vi "Compose TOML String.vi"(8 "error in (no error)":errorcluster, 11 "Value":T1) -> (0 "error out":errorcluster, 3 "String":string)   [LabVIEW 2017, in "TOML.lvlib"]
uses:
  TOML.lvlib
  TOML Value.ctl
  Compose Data.ctl
  Value.ctl
  Value Type.ctl
  Key-Value Pair.ctl
  <vilib>/ErrorRing/Error Ring.xnode
  <vilib>/regexp/Match Regular Expression.xnode
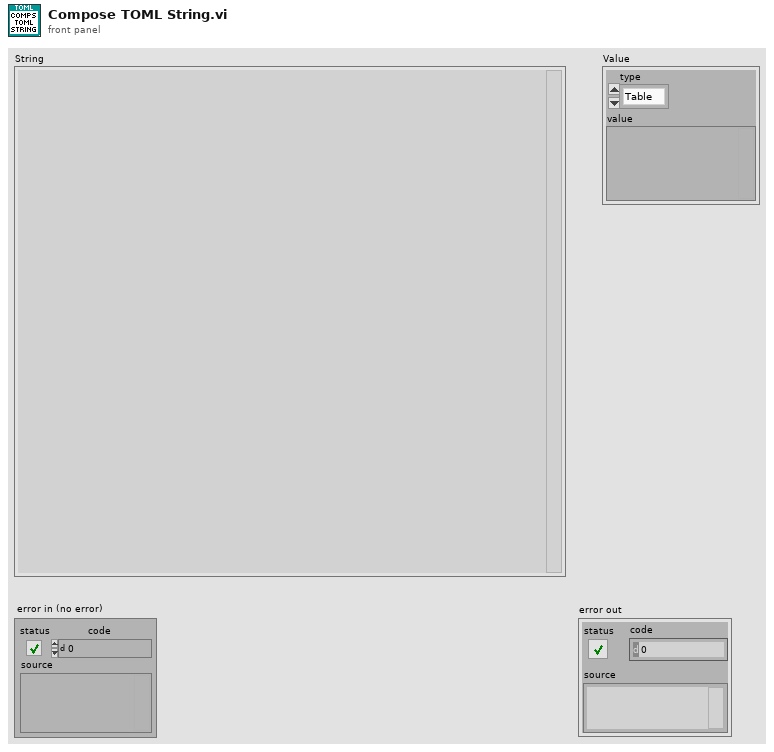
[diagram p1: front panel]
types:
  T1 = typedef "TOML.lvlib/TOML Value.ctl" = cluster{"type":enum16{"Table", "Array", "String", "Integer", "Float", "Boolean", "Offset Date-Time", "Local Date-Time", "Local Date", "Local Time", "Path"}, "value":variant}
  T2 = typedef "TOML.lvlib/Compose Data.ctl" = cluster{"Value":T3, "Prepend":string, "Append":string, "Inline":bool, "Name":string}
  T3 = typedef "TOML.lvlib/Value.ctl" = cluster{"Type":T4, "Value":variant}
  T4 = typedef "TOML.lvlib/Value Type.ctl" = enum16{"Table", "Array", "String", "Integer", "Float", "Boolean", "Offset Date-Time", "Local Date-Time", "Local Date", "Local Time", "Path"}
  T5 = typedef "TOML.lvlib/Key-Value Pair.ctl" = cluster{"Key":string, "Value":T3}
  T6 = enum16{"Table", "Array", "String", "Integer", "Float", "Boolean", "Offset Date-Time", "Local Date-Time", "Local Date", "Local Time"}
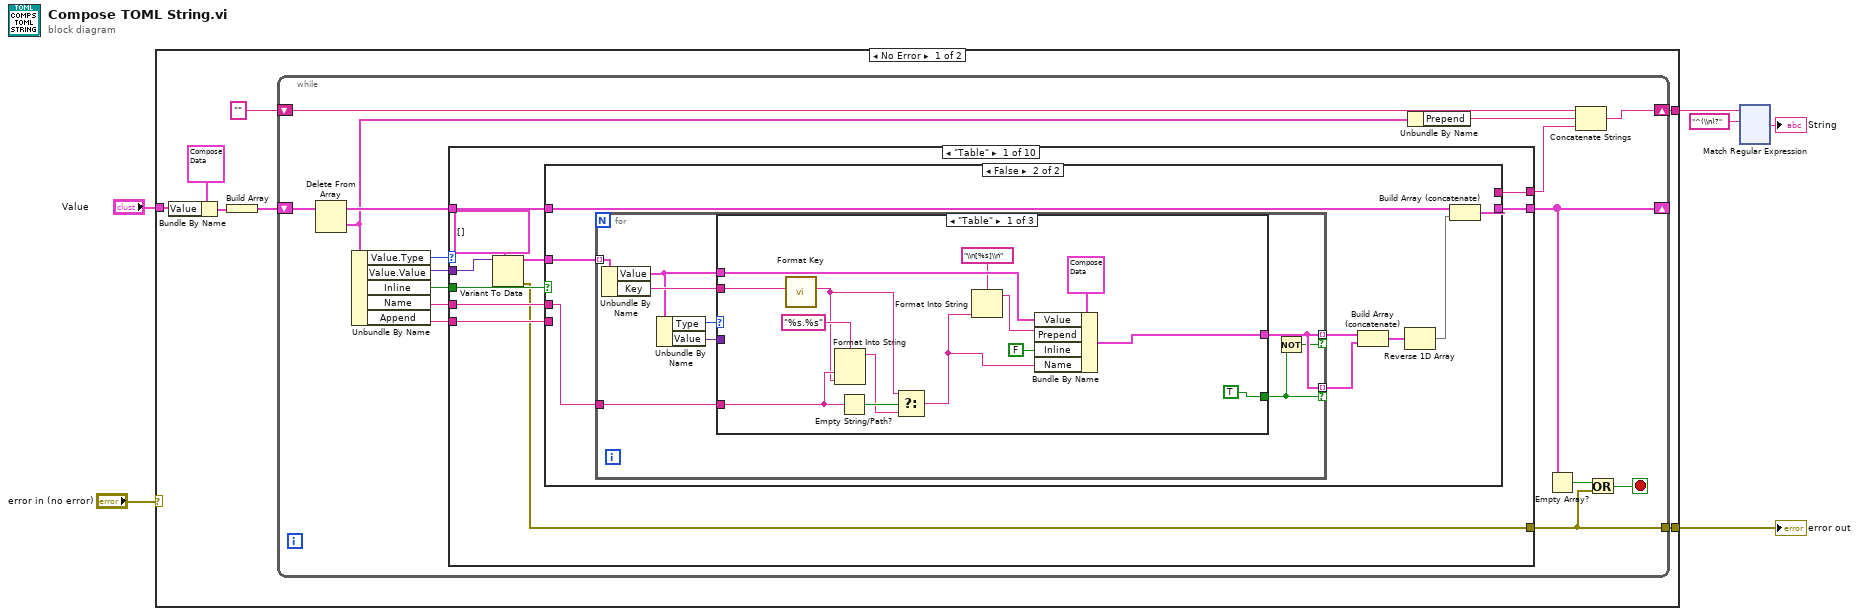
[diagram p0: block diagram]
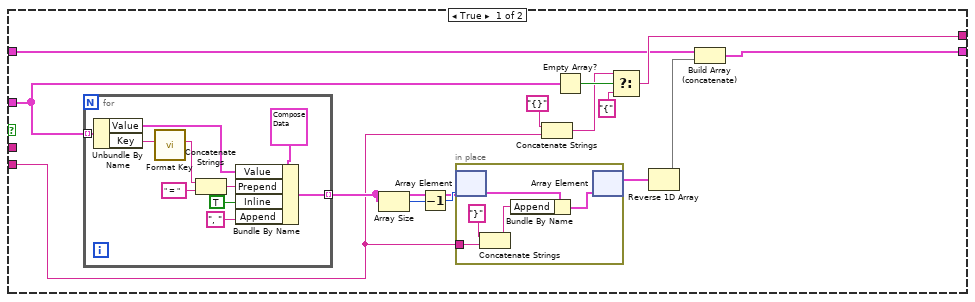
[diagram p2: hidden frame]
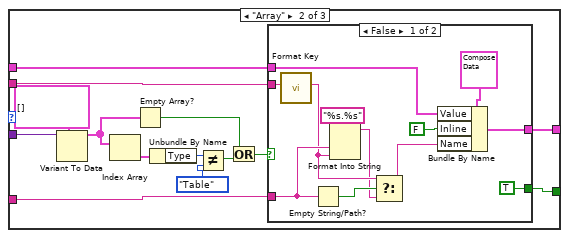
[diagram p3: hidden frame]
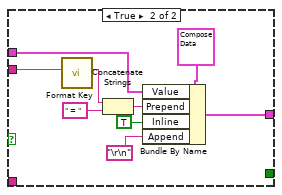
[diagram p4: hidden frame]
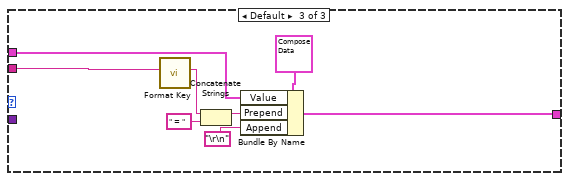
[diagram p5: hidden frame]
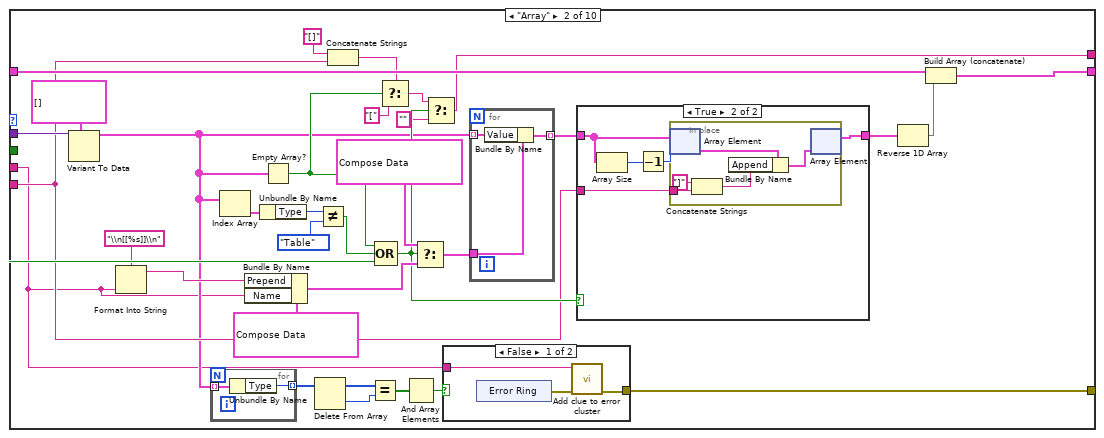
[diagram p6: hidden frame]
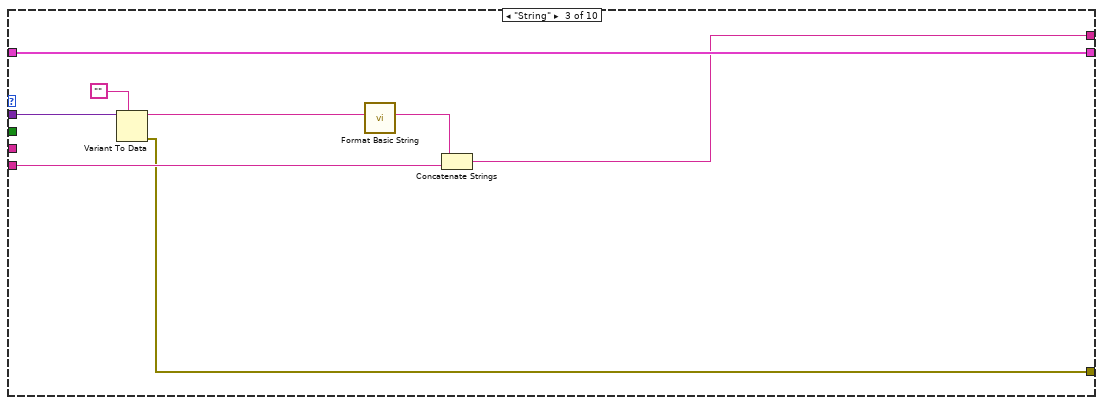
[diagram p9: hidden frame]
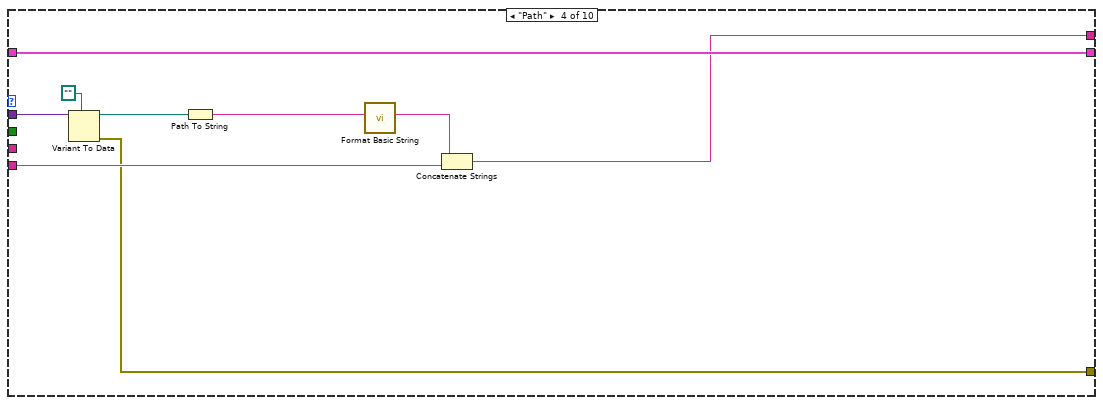
[diagram p10: hidden frame]
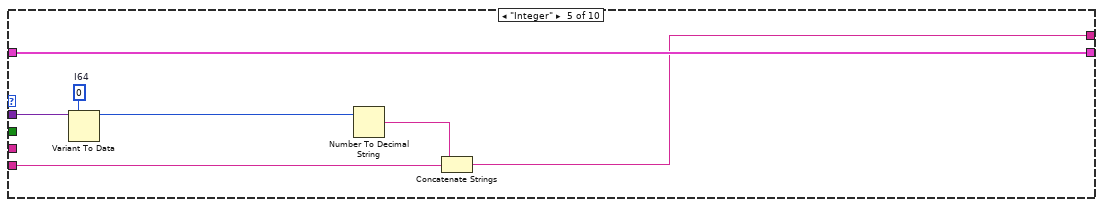
[diagram p11: hidden frame]
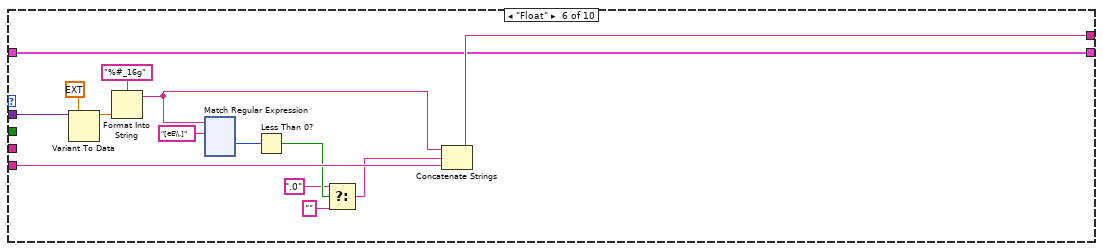
[diagram p12: hidden frame]
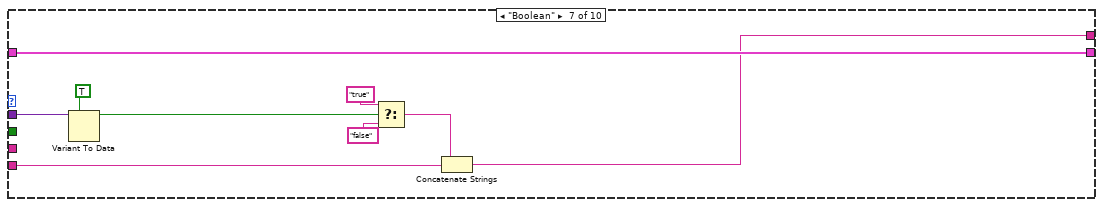
[diagram p13: hidden frame]
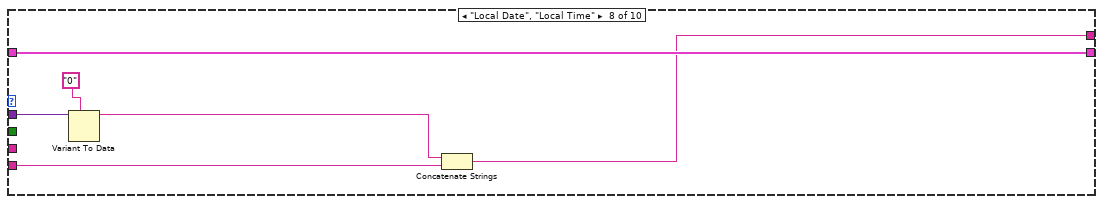
[diagram p14: hidden frame]
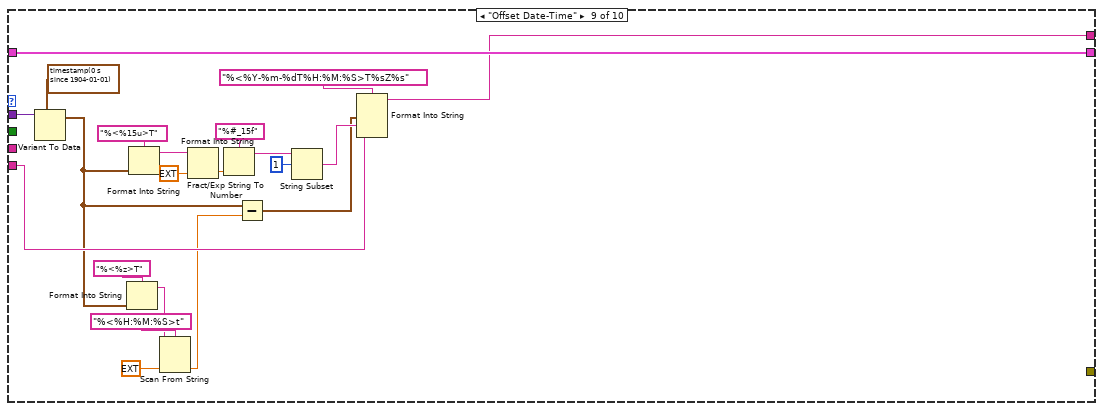
[diagram p15: hidden frame]
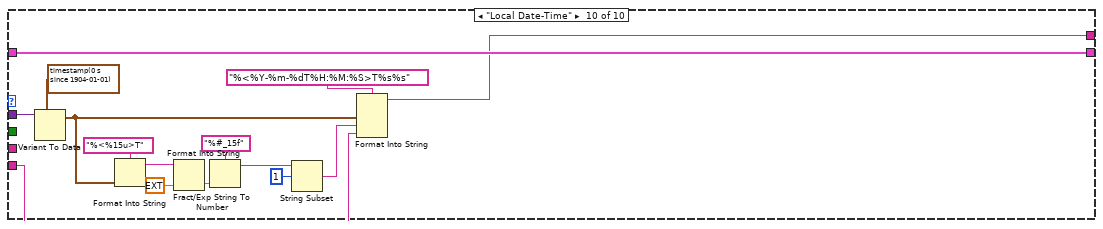
[diagram p16: hidden frame]
diagram:
  n1 = case shown="No Error" "error in (no error)" {
    selector: "error in (no error)" -> [_ w401]
    tunnel: "Value" -> [w10 _]
    tunnel: [w8 _] -> w1
    tunnel: [w7 w401] -> w4
    frame No Error {
      n2 = Bundle By Name(cluster=T2 {"Value"={"Type"=enum."Table", "Value"=variant}, "Prepend"="", "Append"="", "Inline"=FALSE, "Name"=""}, "Value"=w10) -> (w9:T2)
      n3 = Build Array(w9) -> (w12:T2[])
      n4 = while {
        shift-right: [w20] -> w8
        shift-left: "" -> [w23]
        shift-right: [w21] -> _
        shift-left: w12 -> [w29]
        tunnel: [w14] -> w7
        stop <- w15 stop-if-true
        n5 = Delete From Array(array=w29) -> (deleted portion=w18:T2, array with subset deleted=w26:T2[])  [unwired: 2 in]
        n6 = Unbundle By Name(w18) -> ("Value.Type"=w28:T4, "Value.Value"=w27:variant, "Inline"=w25:bool, "Name"=w24:string, "Append"=w16:string)
        n7 = case shown="\"Table\"" w28 {
          tunnel: w27 -> [w36 w177 w204 w213 w220 w235 w358 w364 w384 w399]
          tunnel: w26 -> [w39 w164 w205 w214 w221 w230 w356 w362 w385 w400]
          tunnel: [w38 w151 w205 w214 w221 w230 w356 w362 w385 w400] -> w21
          tunnel: w25 -> [w37 w171 _ _ _ _ _ _ _ _]
          tunnel: w24 -> [w31 w143 _ _ _ _ _ _ _ _]
          tunnel: [w32 w157 w200 w209 w215 w232 w350 w359 w376 w393] -> w19
          tunnel: w16 -> [w33 w152 w201 w210 w218 w233 w357 w363 w377 w394]
          tunnel: [w30 w145 w198 w206 _ _ _ _ _ _] -> w14
          frame "Table" {
            n8 = Variant To Data(type=T5[] [], Variant=w36) -> (data=w34:T5[], error out=w30:errorcluster)  [unwired: 1 in]
            n9 = case shown="False" w37 {
              tunnel: w39 -> [w43 w76]
              tunnel: [w42 w75] -> w38
              tunnel: w34 -> [w50 w72]
              tunnel: w31 -> [_ w74]
              tunnel: w33 -> [w47 _]
              tunnel: [w46 _] -> w32
              frame True {
                n10 = for {
                  tunnel: w50 -> [w68] mode=indexing
                  tunnel: [w60] -> w51 mode=indexing
                  n11 = Unbundle By Name(w68) -> ("Value"=w65:T3, "Key"=w67:string)
                  n12 = call "Format Key.vi"("Key String"=w67) -> ("Formatted Key"=w63:string)  [unwired: 10 in]
                  n13 = Concatenate Strings(w63, " = " ("string")) -> (w64:string)
                  n14 = Bundle By Name(cluster=T2 {"Value"={"Type"=enum."Table", "Value"=variant}, "Prepend"="", "Append"="", "Inline"=FALSE, "Name"=""}, "Value"=w65, "Prepend"=w64, "Inline"=TRUE, "Append"=", ") -> (w60:T2)
                }
                n15 = Array Size(array=w51) -> (size(s)=w53:i32)
                n16 = Decrement(x=w53) -> (x-1=w52:i32)
                n17 = in-place {
                  in-place-border: w47 -> [w54]
                  n18 = in-place-array #1(w51, w52) -> (w58:T2)
                  n19 = Concatenate Strings("}" ("Prepend"), w54) -> (w55:string)
                  n20 = Bundle By Name(cluster=w58, "Append"=w55) -> (w57:T2)
                  n21 = in-place-array #1(w57) -> (w45:T2[])  [unwired: 1 out]
                }
                n22 = Concatenate Strings("{}" ("Prepend"), w47) -> (w40:string)
                n23 = Empty Array?(array=w50) -> (empty?=w49:bool)
                n24 = Select(t=w40, s=w49, f="{" ("t")) -> (s? t:f=w46:string)
                n25 = Reverse 1D Array(array=w45) -> (reversed array=w44:T2[])
                n26 = Build Array (concatenate)(w43, w44) -> (w42:T2[])
              }
              frame False {
                n27 = for {
                  tunnel: w72 -> [w85] mode=indexing
                  tunnel: [w79] -> w70 mode=indexing if=w78
                  tunnel: w74 -> [w81]
                  tunnel: [w79] -> w69 mode=indexing if=w77
                  n28 = Unbundle By Name(w85) -> ("Value"=w83:T3, "Key"=w84:string)
                  n29 = Unbundle By Name(w83) -> ("Type"=w82:T4, "Value"=w80:variant)
                  n30 = case shown="\"Table\"" w82 {
                    tunnel: w84 -> [w99 w113 w138]
                    tunnel: [w96 w112 w135] -> w79
                    tunnel: w83 -> [w95 w111 w137]
                    tunnel: w81 -> [w91 w110 _]
                    tunnel: w80 -> [_ w102 _]
                    tunnel: [TRUE w100 _] -> w77
                    frame "Table" {
                      n31 = call "Format Key.vi"("Key String"=w99) -> ("Formatted Key"=w89:string)  [unwired: 10 in]
                      n32 = Format Into String(format string="%s.%s", w91, w89) -> (resulting string=w88:string)  [unwired: 2 in, 1 out]
                      n33 = Empty String/Path?(string/path=w91) -> (empty?=w90:bool)
                      n34 = Select(t=w89, s=w90, f=w88) -> (s? t:f=w87:string)
                      n35 = Format Into String(format string="\\n[%s]\\n", w87) -> (resulting string=w92:string)  [unwired: 2 in, 1 out]
                      n36 = Bundle By Name(cluster=T2 {"Value"={"Type"=enum."Table", "Value"=variant}, "Prepend"="", "Append"="", "Inline"=FALSE, "Name"=""}, "Value"=w95, "Prepend"=w92, "Inline"=FALSE, "Name"=w87) -> (w96:T2)
                    }
                    frame "Array" {
                      n37 = Variant To Data(type=T3[] [], Variant=w102) -> (data=w105:T3[])  [unwired: 1 in, 1 out]
                      n38 = Index Array(array=w105) -> (element=w107:T3)  [unwired: 1 in]
                      n39 = Empty Array?(array=w105) -> (empty?=w109:bool)
                      n40 = Unbundle By Name(w107) -> ("Type"=w106:T4)
                      n41 = Not Equal?(x=w106, y=T6."Table") -> (x != y?=w108:bool)
                      n42 = Or(x=w109, y=w108) -> (x .or. y?=w101:bool)
                      n43 = case shown="False" w101 {
                        tunnel: w113 -> [w120 w128]
                        tunnel: [w123 w126] -> w112
                        tunnel: w111 -> [w122 w129]
                        tunnel: w110 -> [w119 _]
                        tunnel: [TRUE _] -> w100
                        frame False {
                          n44 = call "Format Key.vi"("Key String"=w120) -> ("Formatted Key"=w117:string)  [unwired: 10 in]
                          n45 = Empty String/Path?(string/path=w119) -> (empty?=w118:bool)
                          n46 = Format Into String(format string="%s.%s", w119, w117) -> (resulting string=w116:string)  [unwired: 2 in, 1 out]
                          n47 = Select(t=w117, s=w118, f=w116) -> (s? t:f=w115:string)
                          n48 = Bundle By Name(cluster=T2 {"Value"={"Type"=enum."Table", "Value"=variant}, "Prepend"="", "Append"="", "Inline"=FALSE, "Name"=""}, "Value"=w122, "Inline"=FALSE, "Name"=w115) -> (w123:T2)
                        }
                        frame True {
                          n49 = call "Format Key.vi"("Key String"=w128) -> ("Formatted Key"=w132:string)  [unwired: 10 in]
                          n50 = Concatenate Strings(w132, " = " ("string")) -> (w133:string)
                          n51 = Bundle By Name(cluster=T2 {"Value"={"Type"=enum."Table", "Value"=variant}, "Prepend"="", "Append"="", "Inline"=FALSE, "Name"=""}, "Value"=w129, "Prepend"=w133, "Inline"=TRUE, "Append"="\r\n") -> (w126:T2)
                        }
                      }
                    }
                    frame Default {
                      n52 = call "Format Key.vi"("Key String"=w138) -> ("Formatted Key"=w140:string)  [unwired: 10 in]
                      n53 = Concatenate Strings(w140, " = " ("string")) -> (w141:string)
                      n54 = Bundle By Name(cluster=T2 {"Value"={"Type"=enum."Table", "Value"=variant}, "Prepend"="", "Append"="", "Inline"=FALSE, "Name"=""}, "Value"=w137, "Prepend"=w141, "Append"="\r\n") -> (w135:T2)
                    }
                  }
                  n55 = Not(x=w77) -> (.not. x?=w78:bool)
                }
                n56 = Build Array (concatenate)(w70, w69) -> (w71:T2[])
                n57 = Reverse 1D Array(array=w71) -> (reversed array=w73:T2[])
                n58 = Build Array (concatenate)(w76, w73) -> (w75:T2[])
              }
            }
          }
          frame "Array" {
            n59 = Variant To Data(type=T3[] [], Variant=w177) -> (data=w144:T3[])  [unwired: 1 in, 1 out]
            n60 = Format Into String(format string="\\n[[%s]]\\n", w143) -> (resulting string=w154:string)  [unwired: 2 in, 1 out]
            n61 = for {
              tunnel: w144 -> [w183] mode=indexing
              tunnel: [w182] -> w150 mode=indexing
              n62 = Unbundle By Name(w183) -> ("Type"=w182:T4)
            }
            n63 = Index Array(array=w144) -> (element=w175:T3)  [unwired: 1 in]
            n64 = Bundle By Name(cluster=T2 {"Value"={"Type"=enum."Table", "Value"=variant}, "Prepend"="", "Append"="", "Inline"=FALSE, "Name"=""}, "Prepend"=w154, "Name"=w143) -> (w168:T2)
            n65 = Unbundle By Name(w175) -> ("Type"=w174:T4)
            n66 = Empty Array?(array=w144) -> (empty?=w161:bool)
            n67 = Delete From Array(array=w150) -> (deleted portion=w148:T4, array with subset deleted=w149:T4[])  [unwired: 2 in]
            n68 = Not Equal?(x=w174, y=T6."Table") -> (x != y?=w172:bool)
            n69 = Concatenate Strings("[]", w152) -> (w159:string)
            n70 = Equal?(x=w149, y=w148) -> (x = y?=w147:bool[])
            n71 = Compound Arithmetic op=OR(w161, w172, w171) -> (w158:bool)
            n72 = Select(t=w159, s=w161, f="[") -> (s? t:f=w156:string)
            n73 = And Array Elements(Boolean array=w147) -> (logical AND=w146:bool)
            n74 = Select(t=T2 {"Value"={"Type"=enum."Table", "Value"=variant}, "Prepend"="", "Append"=", ", "Inline"=TRUE, "Name"=""} ("cluster"), s=w158, f=w168) -> (s? t:f=w167:T2)
            n75 = Select(t=w156, s=w158, f="") -> (s? t:f=w157:string)
            n76 = case shown="False" w146 {
              tunnel: [w179 _] -> w145
              tunnel: w143 -> [w178 _]
              frame False {
                n77 = xnode "Error Ring"() -> ("error out"=w180:errorcluster)
                n78 = call "Add clue to error cluster.vi"("error in (no error)"=w180, "String"=w178) -> ("error out"=w179:errorcluster)  [unwired: 9 in]
              }
              frame True {
              }
            }
            n79 = for {
              tunnel: w144 -> [w197] mode=indexing
              tunnel: w167 -> [w196]
              tunnel: [w195] -> w166 mode=indexing
              n80 = Bundle By Name(cluster=w196, "Value"=w197) -> (w195:T2)
            }
            n81 = case shown="True" w158 {
              tunnel: w166 -> [w184 w186]
              tunnel: [w184 w187] -> w165
              tunnel: w152 -> [_ w185]
              frame False {
              }
              frame True {
                n82 = Array Size(array=w186) -> (size(s)=w189:i32)
                n83 = Decrement(x=w189) -> (x-1=w188:i32)
                n84 = in-place {
                  in-place-border: w185 -> [w190]
                  n85 = in-place-array #2(w186, w188) -> (w194:T2)
                  n86 = Concatenate Strings("]" ("string"), w190) -> (w192:string)
                  n87 = Bundle By Name(cluster=w194, "Append"=w192) -> (w193:T2)
                  n88 = in-place-array #2(w193) -> (w187:T2[])  [unwired: 1 out]
                }
              }
            }
            n89 = Reverse 1D Array(array=w165) -> (reversed array=w163:T2[])
            n90 = Build Array (concatenate)(w164, w163) -> (w151:T2[])
          }
          frame "String" {
            n91 = Variant To Data(type="", Variant=w204) -> (data=w203:string, error out=w198:errorcluster)  [unwired: 1 in]
            n92 = call "Format Basic String.vi"("String"=w203) -> ("Formatted Basic String"=w202:string)  [unwired: 10 in]
            n93 = Concatenate Strings(w202, w201) -> (w200:string)
          }
          frame "Path" {
            n94 = Variant To Data(type=path "", Variant=w213) -> (data=w212:path, error out=w206:errorcluster)  [unwired: 1 in]
            n95 = Path To String(path=w212) -> (string=w207:string)
            n96 = call "Format Basic String.vi"("String"=w207) -> ("Formatted Basic String"=w211:string)  [unwired: 10 in]
            n97 = Concatenate Strings(w211, w210) -> (w209:string)
          }
          frame "Integer" {
            w219 = i64 0  # I64
            n98 = Variant To Data(type=w219, Variant=w220) -> (data=w217:i64)  [unwired: 1 in, 1 out]
            n99 = Number To Decimal String(number=w217) -> (decimal integer string=w216:string)  [unwired: 1 in]
            n100 = Concatenate Strings(w216, w218) -> (w215:string)
          }
          frame "Float" {
            n101 = Variant To Data(type=ext 0.0, Variant=w235) -> (data=w231:ext)  [unwired: 1 in, 1 out]
            n102 = Format Into String(format string="%#_16g", w231) -> (resulting string=w225:string)  [unwired: 2 in, 1 out]
            n103 = xnode "Match Regular Expression"("input string"=w225, "regular expression"="[eE\\.]") -> ("offset past match"=w227:i32)  [unwired: 4 in, 4 out]
            n104 = Less Than 0?(x=w227) -> (x < 0?=w226:bool)
            n105 = Select(t=".0", s=w226, f="") -> (s? t:f=w222:string)
            n106 = Concatenate Strings(w225, w222, w233) -> (w232:string)
          }
          frame "Boolean" {
            n107 = Variant To Data(type=TRUE, Variant=w358) -> (data=w354:bool)  [unwired: 1 in, 1 out]
            n108 = Select(t="true", s=w354, f="false") -> (s? t:f=w351:string)
            n109 = Concatenate Strings(w351, w357) -> (w350:string)
          }
          frame "Local Date", "Local Time" {
            n110 = Variant To Data(type="0", Variant=w364) -> (data=w360:string)  [unwired: 1 in, 1 out]
            n111 = Concatenate Strings(w360, w363) -> (w359:string)
          }
          frame "Offset Date-Time" {
            n112 = Variant To Data(type=timestamp(0 s since 1904-01-01), Variant=w384) -> (data=w366:timestamp)  [unwired: 1 in, 1 out]
            n113 = Format Into String(format string="%<%z>T", w366) -> (resulting string=w369:string)  [unwired: 2 in, 1 out]
            n114 = Format Into String(format string="%<%15u>T", w366) -> (resulting string=w374:string)  [unwired: 2 in, 1 out]
            n115 = Scan From String(format string="%<%H:%M:%S>t", input string=w369, default 1=ext 0.0 ("default value 1")) -> (output 1=w367:ext)  [unwired: 2 in, 3 out]
            n116 = Fract/Exp String To Number(string=w374, default (0 dbl)=ext 0.0 ("default (0 DBL)")) -> (number=w372:ext)  [unwired: 2 in, 1 out]
            n117 = Format Into String(format string="%#_15f", w372) -> (resulting string=w381:string)  [unwired: 2 in, 1 out]
            n118 = Subtract(x=w366, y=w367) -> (x-y=w365:timestamp)
            n119 = String Subset(string=w381, offset (0)=1) -> (substring=w378:string)  [unwired: 1 in]
            n120 = Format Into String(format string="%<%Y-%m-%dT%H:%M:%S>T%sZ%s", w365, w378, w377) -> (resulting string=w376:string)  [unwired: 2 in, 1 out]
          }
          frame "Local Date-Time" {
            n121 = Variant To Data(type=timestamp(0 s since 1904-01-01), Variant=w399) -> (data=w386:timestamp)  [unwired: 1 in, 1 out]
            n122 = Format Into String(format string="%<%15u>T", w386) -> (resulting string=w390:string)  [unwired: 2 in, 1 out]
            n123 = Fract/Exp String To Number(string=w390, default (0 dbl)=ext 0.0 ("default (0 DBL)")) -> (number=w388:ext)  [unwired: 2 in, 1 out]
            n124 = Format Into String(format string="%#_15f", w388) -> (resulting string=w387:string)  [unwired: 2 in, 1 out]
            n125 = String Subset(string=w387, offset (0)=1) -> (substring=w395:string)  [unwired: 1 in]
            n126 = Format Into String(format string="%<%Y-%m-%dT%H:%M:%S>T%s%s", w386, w395, w394) -> (resulting string=w393:string)  [unwired: 2 in, 1 out]
          }
        }
        n127 = Unbundle By Name(w18) -> ("Prepend"=w17:string)
        n128 = Empty Array?(array=w21) -> (empty?=w22:bool)
        n129 = Concatenate Strings(w23, w17, w19) -> (w20:string)
        n130 = Or(x=w22, y=w14) -> (x .or. y?=w15:bool)
      }
    }
    frame Error {
    }
  }
  "error out" <- w4
  n131 = xnode "Match Regular Expression"("input string"=w1, "regular expression"="^(\\n)?") -> ("after match"=→"String":string)  [unwired: 4 in, 4 out]
